vi "ppm.vi"() -> ()   [LabVIEW 2021]
uses:
  <vilib>/measure/mamon.llb/Trigger Detection for 1 Channel (obs).vi
  <vilib>/measure/NI_MABase.lvlib
  Instance           4 13Saved   PPM-1 .vi
  <vilib>/measure/NI_MAPro.lvlib
panel:
  in  "duty cycle (%)":dbl=12.5 min=2.5 max=25.0 format="%0.2f"
  in  "Servo Position":dbl=49.205873713538864
  out "Demodulated signal":dbl(graph)=612.0
  out "PPM output":waveform(dbl)(graph)={"t0"=timestamp(0 s since 1904-01-01), "dt"=1e-05, "Y"=array[100000 elements]}
  in  "stop":bool
  # "PULSE POSITION MODULATION & DEMODULATION"
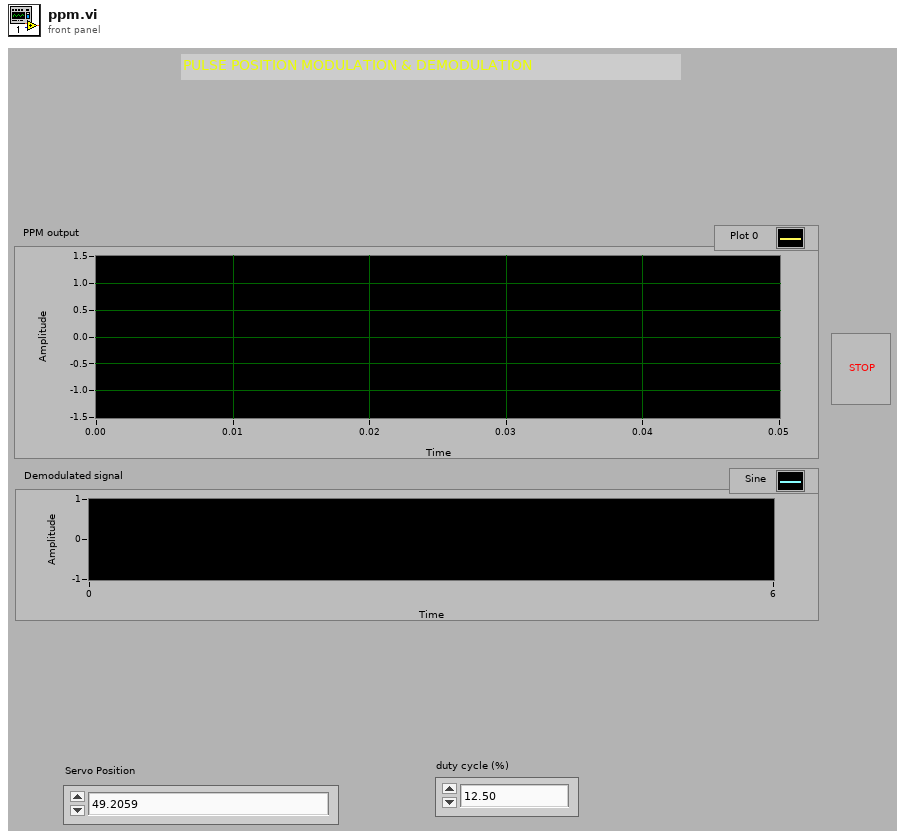
[diagram p1: front panel]
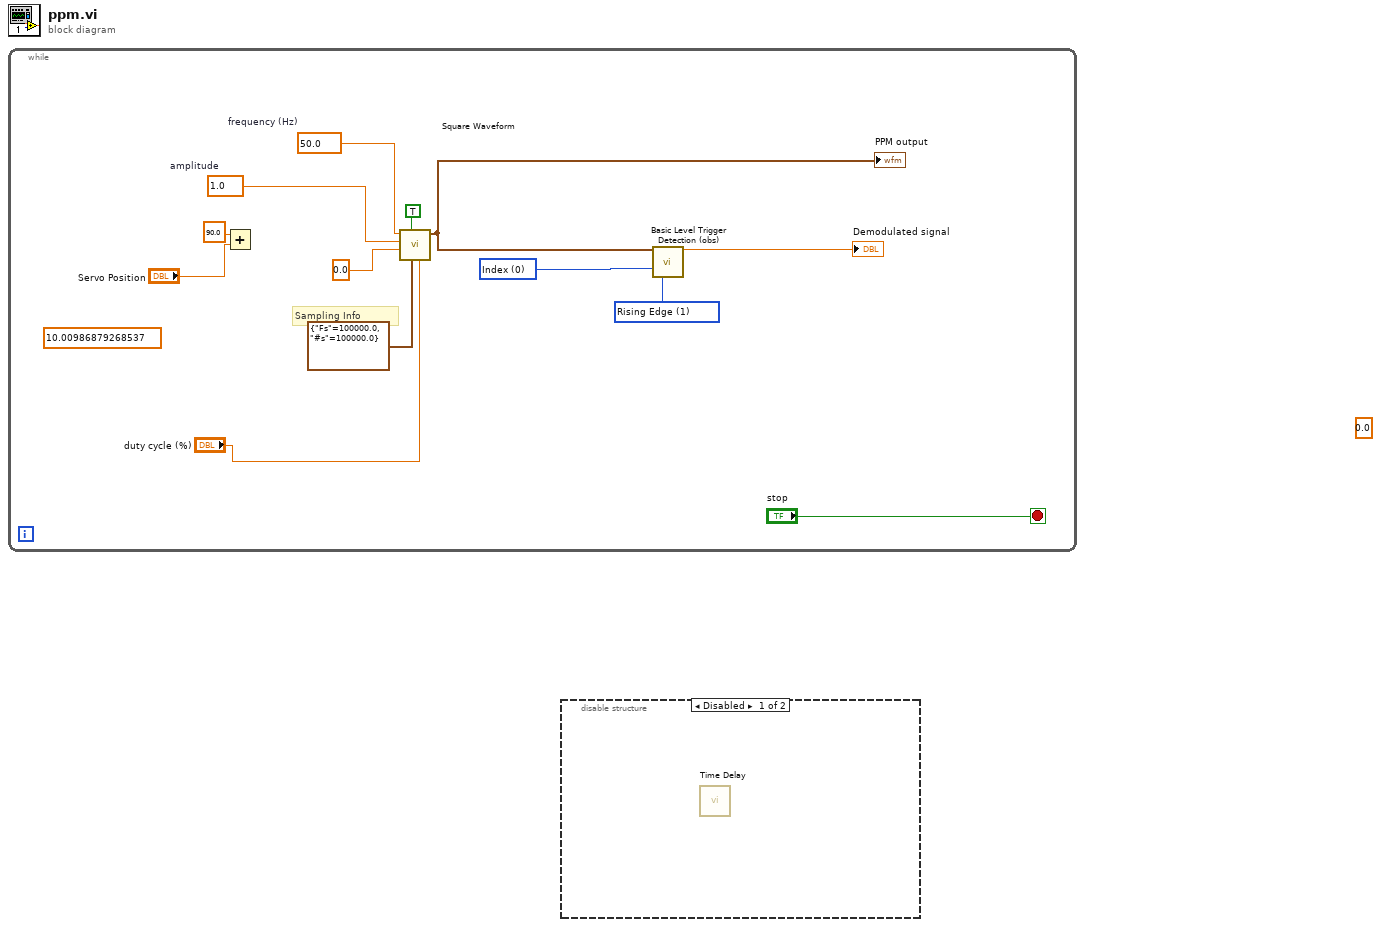
[diagram p0: block diagram]
diagram:
  (unwired) 0.0 ("Waveform Chart")
  n1 = while {
    stop <- "stop" stop-if-true
    (unwired) 10.00986879268537 ("Servo Position")
    w6 = u16 0 items=["Index", "Time"] ("mode")
    w7 = u16 1 items=["Falling Edge", "Rising Edge"] ("slope")
    w13 = 50.0  # frequency (Hz)
    w12 = 1.0  # amplitude
    # "Sampling Info"
    n2 = Add(x=90.0, y="Servo Position") -> ()  [unwired: 1 out]
    n3 = call <vilib>:"Square Waveform.vi"("duty cycle (%)"="duty cycle (%)", "sampling info"=cluster{"Fs":dbl, "#s":dbl} {"Fs"=100000.0, "#s"=100000.0}, "reset signal"=TRUE, "phase"=0.0, "amplitude"=w12, "frequency"=w13) -> ("signal out"=w8:waveform(dbl))  [unwired: 4 in, 1 out]
    "PPM output" <- w8
    n4 = call-poly <vilib>:"Basic Level Trigger Detection (obs).vi"("signal in"=w8, "location mode"=w6, "trigger slope"=w7) -> ("trigger location"=→"Demodulated signal":dbl)  [unwired: 10 in, 2 out]
  }
  n5 = disable-structure shown="Disabled" {
    frame Disabled {
      n6 = call "Time Delay"() -> ()  [unwired: 11 in, 1 out]
    }
    frame Enabled {
    }
  }
